vi "1D Slice to 2D.vi"(10 "Fit Range":u32[](array[numeric]), 11 "Data In":dbl[](array[numeric])) -> (1 "Slice Start":u32, 2 "Sliced Data":dbl[](array[numeric]), 3 "Indices":u32[](array[numeric]))   [LabVIEW 2012]
uses:
  <userlib>/_OpenG.lib/array/array.llb/Slice 1D Array (DBL)__ogtk.vi
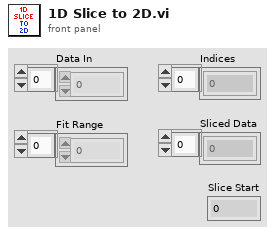
[diagram p1: front panel]
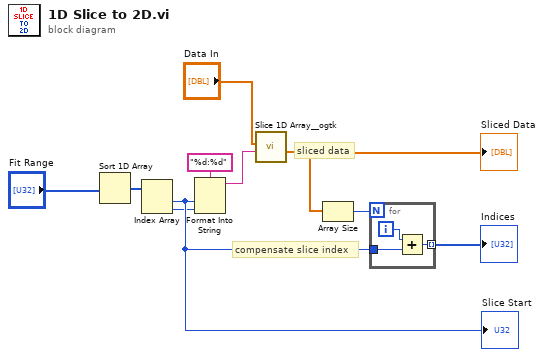
[diagram p0: block diagram]
diagram:
  # "compensate slice index"
  # "sliced data"
  n1 = Sort 1D Array(array="Fit Range") -> (sorted array=w4:u32[])
  n2 = Index Array(array=w4) -> (element #1=w10:u32, element #2=w3:u32)  [unwired: 2 in]
  "Slice Start" <- w10
  n3 = Format Into String(format string="%d:%d", w10, w3) -> (resulting string=w6:string)  [unwired: 2 in, 1 out]
  n4 = call-poly <userlib>:"Slice 1D Array__ogtk.vi"("slice"=w6, "array"="Data In") -> ("subarray (array[i:j])"=w8:dbl[])  [unwired: 5 in]
  "Sliced Data" <- w8
  n5 = Array Size(array=w8) -> (size(s)=w2:i32)
  n6 = for {
    N: w2 -> [_]
    tunnel: [w12] -> w1 mode=indexing
    tunnel: w10 -> [w11]
    i -> [w13]
    n7 = Add(x=w13, y=w11) -> (x+y=w12:u32)
  }
  "Indices" <- w1
